vi "Set plot cursor snap-to-plot and colour.vi"(9 "Data In":T1, 11 "Waveform Graph in":T6) -> (3 "WaveformGraph out":T6)   [LabVIEW 2013, in "XGrapher.xctl"]
uses:
  XGrapher.xctl
  Typedefs/Xctrl-Waveform graph ref.ctl
  Data 1.ctl
  Typedefs/Xctrl-Data array.ctl
  Typedefs/Xcrtl-Data format definition.ctl
  Typedefs/Xctl-XY data type definition.ctl
  Typedefs/Xctrl-ROI type enum.ctl
panel:
  out "Selected POI index":u16
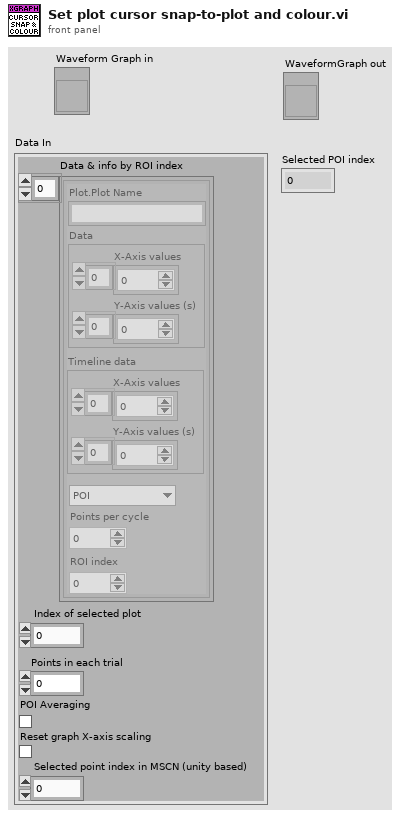
[diagram p1: front panel]
types:
  T1 = typedef "XGrapher.xctl/Data 1.ctl" = cluster{"Data & info by ROI index":T2, "Index of selected plot":u16, "Points in each trial":i32, "POI Averaging":bool, "Reset graph X-axis scaling":bool, "Selected point index in MSCN (unity based)":u16}
  T2 = typedef "Xctrl-Data array.ctl" = T3[]
  T3 = typedef "XGrapher.xctl/Xcrtl-Data format definition.ctl" = cluster{"Plot.Plot Name":string, "Data":T4, "Timeline data":T4, "Type":T5, "Points per cycle":u16, "ROI index":u16}
  T4 = typedef "XGrapher.xctl/Xctl-XY data type definition.ctl" = cluster{"X-Axis values":sgl[], "Y-Axis values (s)":i32[]}
  T5 = typedef "Xctrl-ROI type enum.ctl" = enum16{"POI", "Mini-scan", "Group"}
  T6 = typedef "XGrapher.xctl/Xctrl-Waveform graph ref.ctl" = refnum<vi>
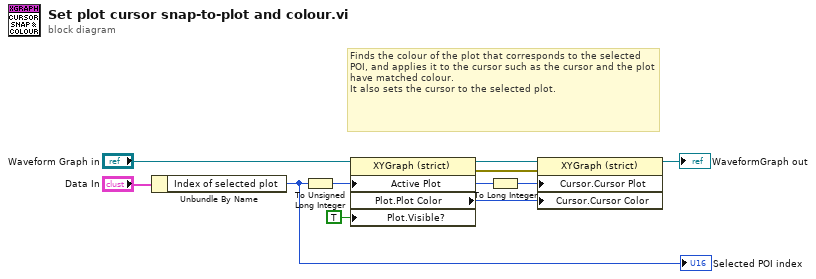
[diagram p0: block diagram]
diagram:
  # "Finds the colour of the plot that corresponds to the selected POI, and applies it to the cursor such as the cursor and the plot have matched colour.\nIt also sets the cursor to the selected plot."
  n1 = Unbundle By Name("Data In") -> ("Index of selected plot"=w2:u16)
  "Selected POI index" <- w2
  n2 = To Unsigned Long Integer(number=w2) -> (unsigned 32bit integer=w8:u32)
  n3 = property on="Get Plot's Color" class="XYGraph (strict)"(reference="Waveform Graph in", "Active Plot"=w8, "Plot.Visible?"=TRUE ("Plot.Visible")) -> (reference out=w5:T6, error out=w6:errorcluster, "Plot.Plot Color"=w7:u32)  [unwired: 1 in]
  n4 = To Long Integer(number=w8) -> (32bit integer=w9:i32)
  n5 = property on="Get Plot's Color" class="XYGraph (strict)"(reference=w5, error in=w6, "Cursor.Cursor Plot"=w9, "Cursor.Cursor Color"=w7) -> (reference out=→"WaveformGraph out":T6)  [unwired: 1 out]
